vi "Host.vi"() -> ()   [LabVIEW 2019]
uses:
  <vilib>/Analysis/7linalg.llb/Eigenvalue and Vectors Output Option.ctl
  <vilib>/Analysis/baseanly.llb/Matrix Type of Inverse Matrix.ctl
  <vilib>/Analysis/7linalg.llb/Real Generalized Eigenvalues and Vectors.vi
  <vilib>/Analysis/7linalg.llb/Real Cholesky Factorization.vi
  <vilib>/Analysis/baseanly.llb/Full Cholesky Factorization.vi
  <vilib>/Analysis/baseanly.llb/Full Real Matrix Cholesky Factorization.vi
  <vilib>/FPGAPlugInAG/PXIe-7915/niLvFpga_Open_PXIe-7915.vi
  <vilib>/rvi/interface/common/dynamic/niFpgaDynamicAddResources.vi
  <vilib>/Analysis/baseanly.llb/Real Inverse Matrix.vi
  <vilib>/Analysis/Matrix/Numeric/Multiply/Multiply - RM,RM.vi
  <vilib>/Analysis/7linalg.llb/Real Eigenvalues and Vectors.vi
  <vilib>/Analysis/Matrix/Numeric/Add/Add - RM,RM.vi
  <vilib>/Utility/error.llb/Error Cluster From Error Code.vi
  <vilib>/rvi/errors/niLvFpgaAdjustHostInterfaceError.vi
  <vilib>/FPGAPlugInAG/Dynamic/niLvFpga_Run_Dynamic.vi
  <vilib>/FPGAPlugInAG/Dynamic/niLvFpga_Close_Dynamic.vi
  <vilib>/rvi/interface/nirviOpenFPGA/nirviOpenFPGA.xnode
  FPGA Bitfiles/choleskyfpgav1_FPGATarget_Target_xjOD3-+swO0.lvbitx
  Target.vi
  <vilib>/rvi/interface/nirviMethod/nirviMethod.xnode
  <vilib>/rvi/interface/nirviReadWriteControl/nirviReadWriteControl.xnode
  <vilib>/rvi/interface/nirviCloseFPGA/nirviCloseFPGA.xnode
  <vilib>/Analysis/NI_AALPro.lvlib
  <vilib>/Analysis/NI_AALBase.lvlib
  <vilib>/Analysis/Matrix/NI_Matrix.lvlib
  <vilib>/rvi/errors/niLvFpgaMergeErrorWithErrorCode.vi
  <vilib>/FPGAPlugInAG/Dynamic/niLvFpga_ReadFifo_Dynamic.vi
  <vilib>/FPGAPlugInAG/Dynamic/niLvFpga_WriteFifo_Dynamic.vi
  NiFpgaLv.dll
  <vilib>/rvi/interface/Simulation/niFpgaSimulationCallBeginRW.vi
panel:
  out "T5":u32
  out "T4":u32
  out "T3":u32
  out "T2":u32
  out "T1":u32
  out "Frequencies":dbl[](array[numeric])
  out "Eigenvalues":cdb[][](array[numeric]) format="%#_4g"
  out "Run Time (ms)":u32 format="%_6f"
  out "Elements Remaining 2":u32
  out "Elements Remaining":u32
  out "K input":dbl[][](array[numeric])
  in  "Method":i32(listbox)
  out "M input":dbl[][](array[numeric])
  # "Takes 56 ms to solve without timed loop"
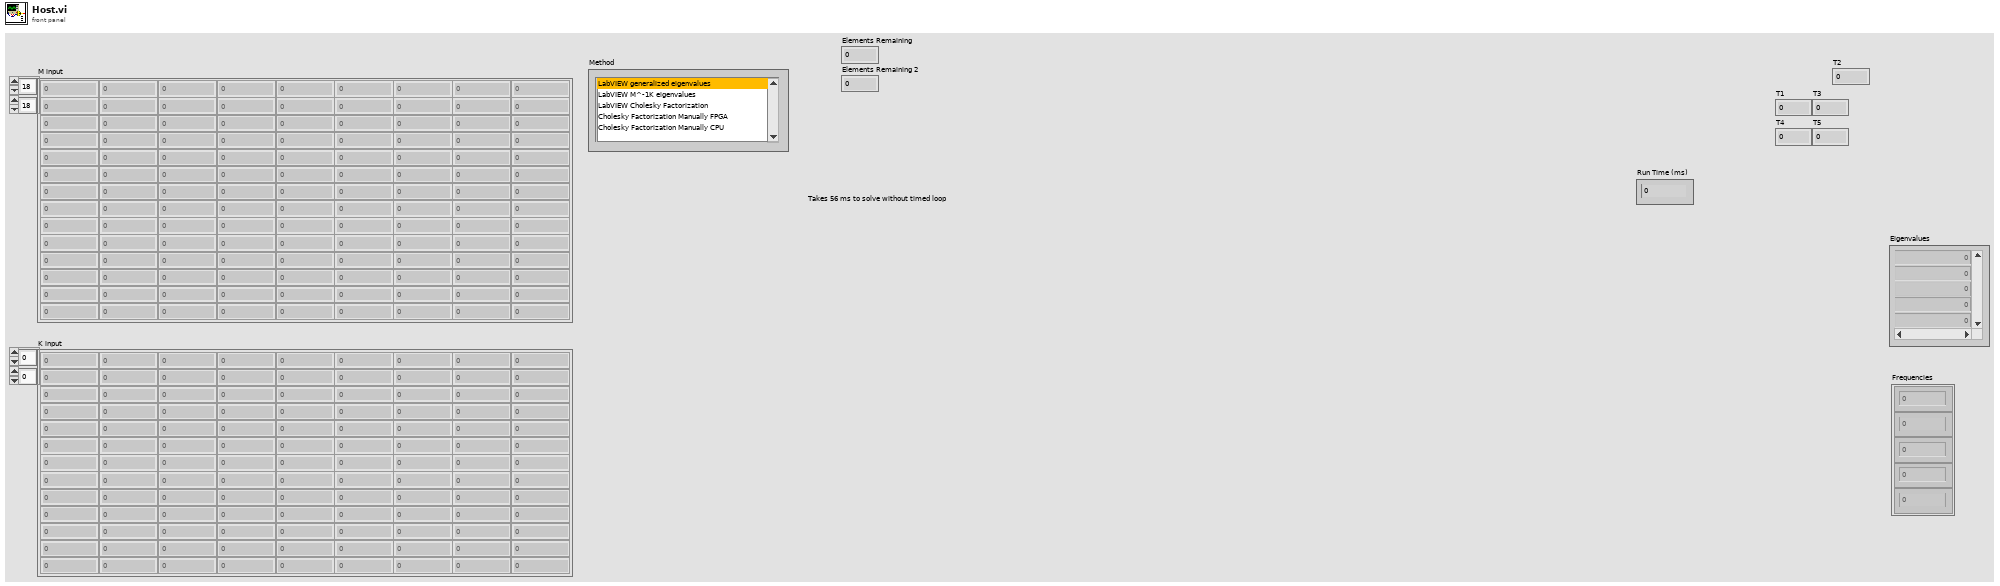
[diagram p1: front panel]
types:
  T1 = typedef "NI_AALBase.lvlib/Matrix Type of Inverse Matrix.ctl" = enum32{"General", "Positive Definite", "Lower Triangular", "Upper Triangular"}
  T2 = typedef "NI_AALPro.lvlib/Eigenvalue and Vectors Output Option.ctl" = i32
  T3 = typedef "NI_Matrix.lvlib/RealMatrix.ctl" = dbl[][]
  T4 = typedef "NI_Matrix.lvlib/ComplexMatrix.ctl" = cdb[][]
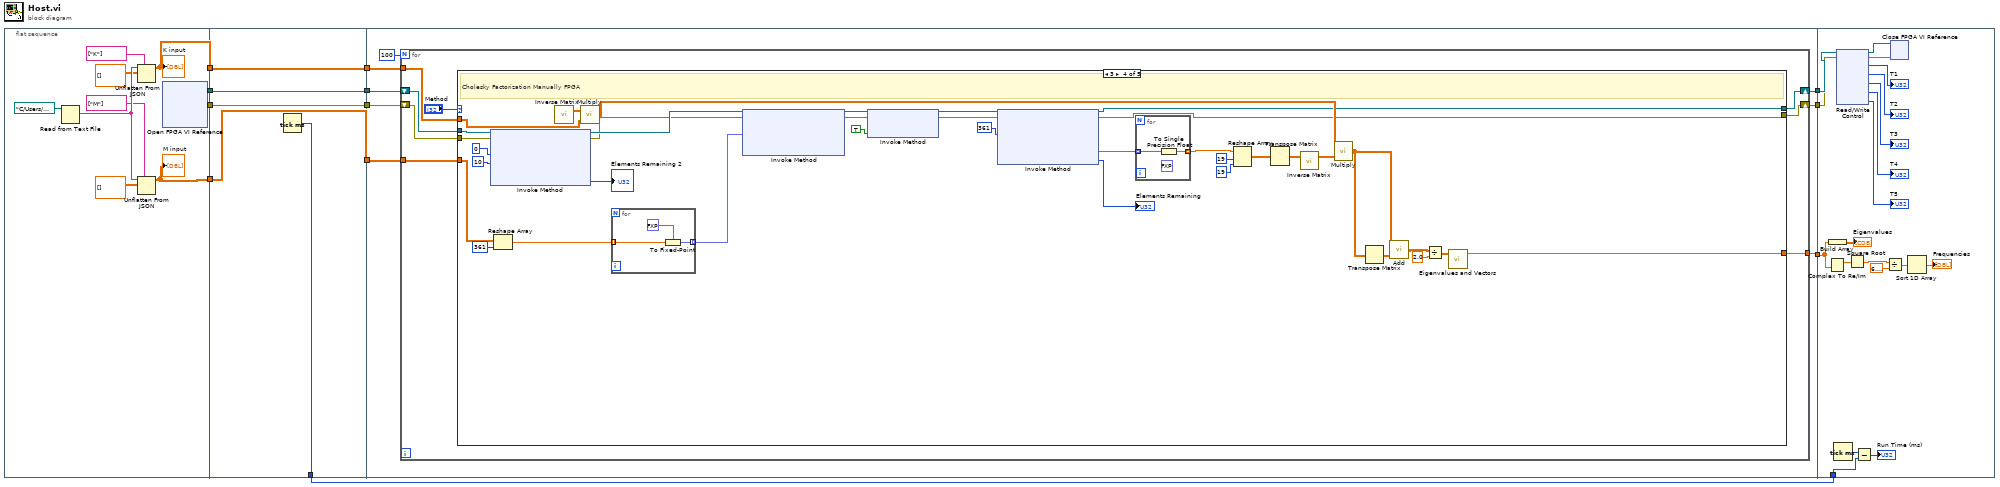
[diagram p0: block diagram]
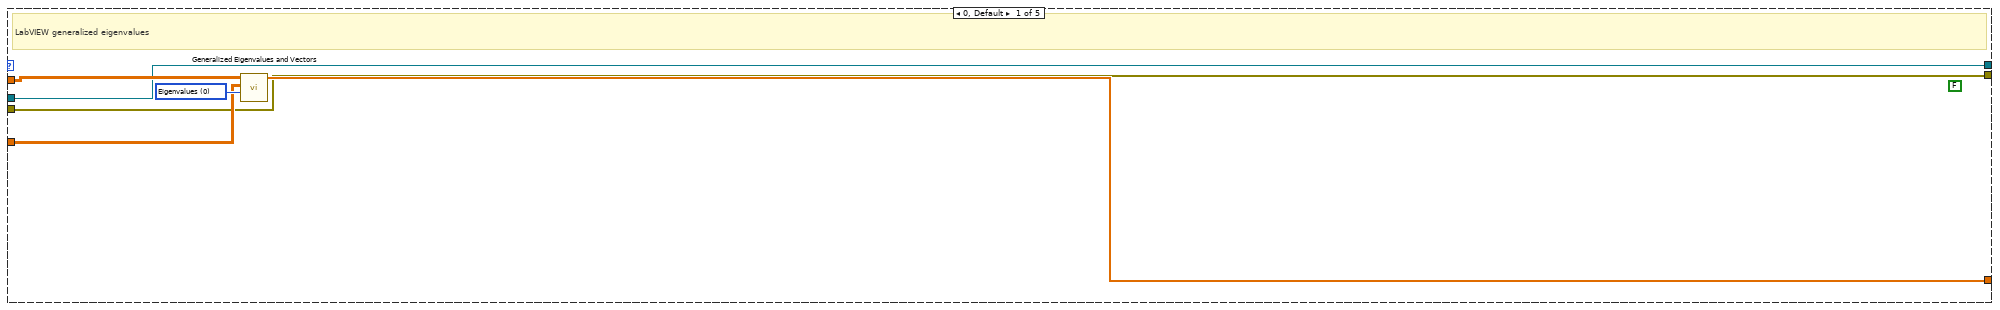
[diagram p2: hidden frame]
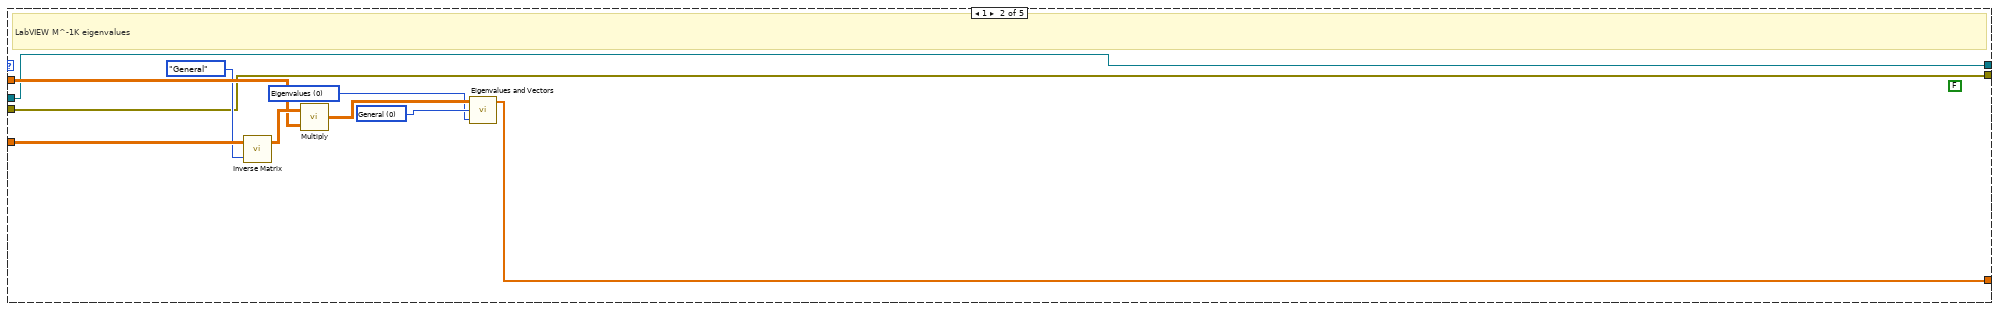
[diagram p3: hidden frame]
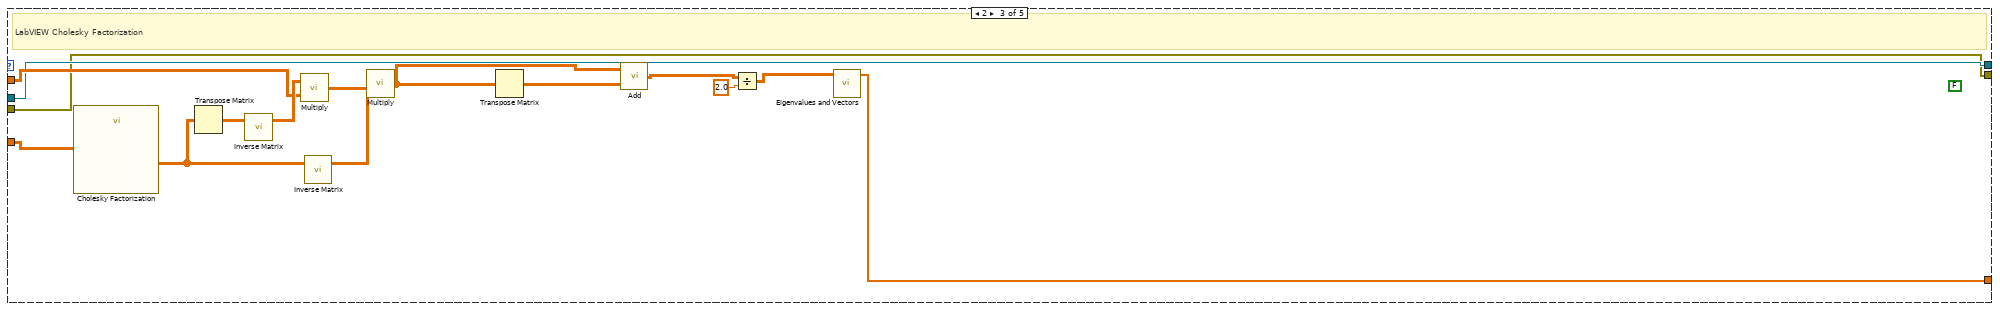
[diagram p4: hidden frame]
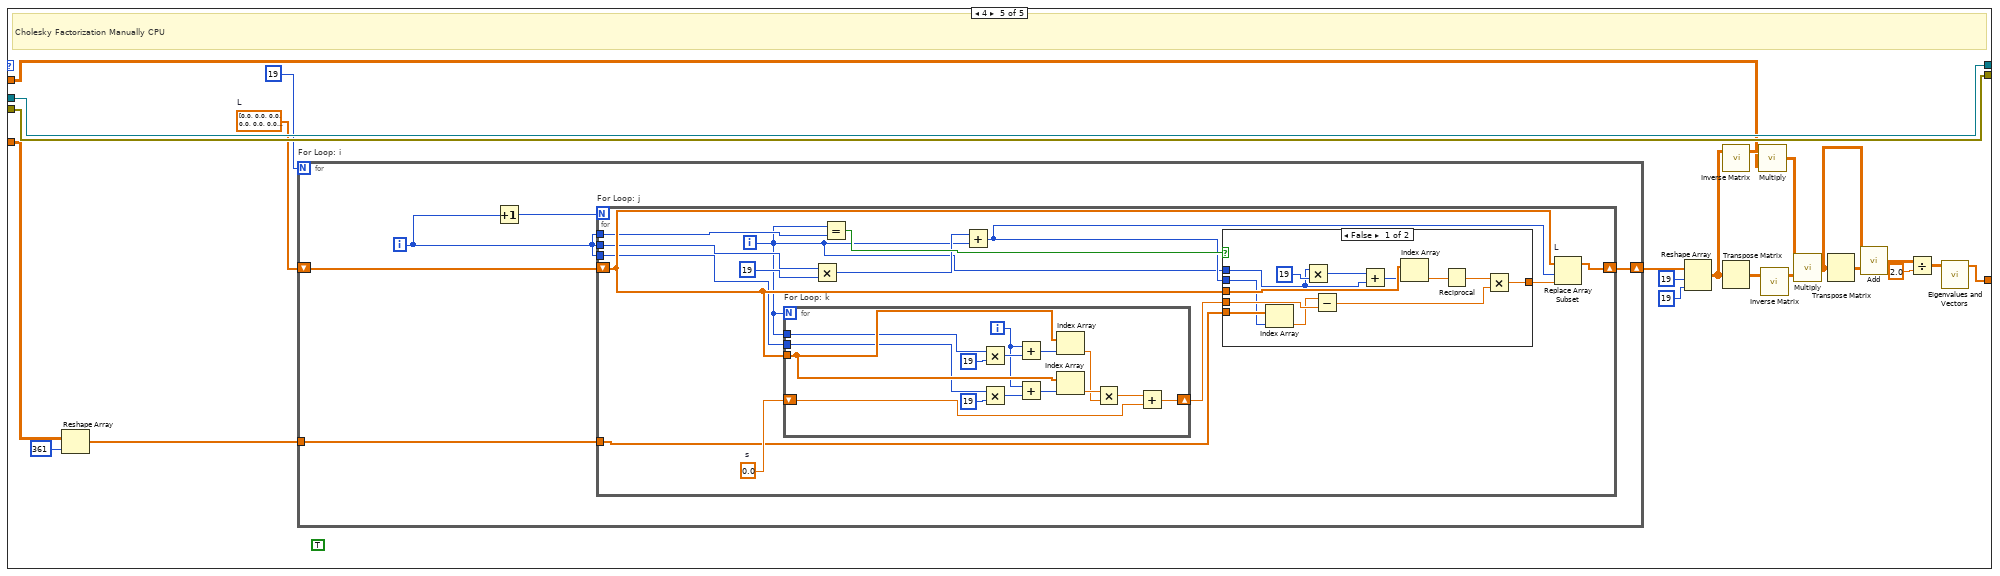
[diagram p5: hidden frame]
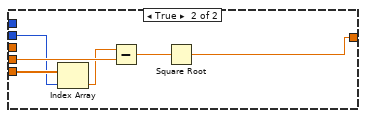
[diagram p6: hidden frame]
diagram:
  n1 = flat-sequence {
    tunnel: [w16] -> w10
    tunnel: [w15] -> w9
    tunnel: [w14] -> w7
    tunnel: [w13] -> w5
    tunnel: [w27] -> w12
    tunnel: [w26] -> w11
    tunnel: [w25] -> w1
    tunnel: w10 -> [w27]
    tunnel: w9 -> [w26]
    tunnel: [w24] -> w8
    tunnel: w7 -> [w24]
    tunnel: [w23] -> w6
    tunnel: w5 -> [w23]
    tunnel: w12 -> [w35]
    tunnel: w11 -> [w34]
    tunnel: w8 -> [w29]
    tunnel: w6 -> [w28]
    tunnel: [w33] -> w4
    tunnel: [w31] -> w3
    tunnel: [w30] -> w2
    tunnel: w4 -> [w196]
    tunnel: w3 -> [w195]
    tunnel: w2 -> [w194]
    tunnel: w1 -> [w193]
    frame #0 {
      n2 = Read from Text File(file (use dialog)=path "C:/Users/PXIe-8880/Documents/AFRL_summer_2019/Cholesky_FPGA/Cholesky_FPGA_V1/data/data.txt") -> (text=w22:string)  [unwired: 3 in, 3 out]
      n3 = Unflatten From JSON(path=string[] ["K"], JSON string=w22, type and defaults=dbl[][] []) -> (value=w15:dbl[][])  [unwired: 4 in, 1 out]
      "K input" <- w15
      n4 = Unflatten From JSON(path=string[] ["M"], JSON string=w22, type and defaults=dbl[][] []) -> (value=w16:dbl[][])  [unwired: 4 in, 1 out]
      "M input" <- w16
      n5 = xnode "Open FPGA VI Reference"() -> ("FPGA VI Reference Out"=w14:refnum<k20>, "error out"=w13:errorcluster)  [unwired: 2 in]
    }
    frame #1 {
      n6 = Tick Count (ms)() -> (millisecond timer value=w25:u32)
    }
    frame #2 {
      n7 = for {
        N: 100 -> [_]
        tunnel: w35 -> [w43]
        tunnel: w34 -> [w42]
        tunnel: [w39] -> w33
        shift-right: [w41] -> w31
        shift-left: w29 -> [w37]
        shift-right: [w40] -> w30
        shift-left: w28 -> [w36]
        n8 = case shown="3" "Method" {
          tunnel: [w48 w55 w68 w95 w116] -> w39
          tunnel: w43 -> [w47 w54 w74 w110 w117]
          tunnel: w42 -> [w46 w53 w70 w96 w118]
          tunnel: w37 -> [w45 w51 w61 w85 w137]
          tunnel: [w45 w51 w61 w89 w137] -> w41
          tunnel: w36 -> [w44 w50 w60 w84 w136]
          tunnel: [w44 w50 w60 w90 w136] -> w40
          frame 0, Default {
            (unwired) FALSE
            w49 = T2 0 items=["Eigenvalues", "Eigenvalues & Vectors"] ("output option")
            # "LabVIEW generalized eigenvalues"
            n9 = call-poly <vilib>:"Generalized Eigenvalues and Vectors.vi"("output option"=w49, "B"=w47, "A"=w46) -> ("Eigenvalues"=w48:cdb[])  [unwired: 3 in, 2 out]
          }
          frame 1 {
            (unwired) FALSE
            w56 = T2 0 items=["Eigenvalues", "Eigenvalues & Vectors"] ("output option")
            w57 = 0 items=["General", "Symmetric"] ("matrix type")
            # "LabVIEW M^-1K eigenvalues"
            n10 = call-poly <vilib>:"Inverse Matrix.vi"("matrix type"=Matrix_Type_of_Inverse_Matrix."General", "Input Matrix"=w54) -> ("Inverse Matrix"=w58:T3)  [unwired: 1 out]
            n11 = call-poly <vilib>:"Multiply.vi"("Real Matrix B"=w53, "Real Matrix A"=w58) -> ("A * B"=w59:T3)
            n12 = call-poly <vilib>:"Eigenvalues and Vectors.vi"("output option"=w56, "matrix type"=w57, "Input Matrix"=w59) -> ("Eigenvalues"=w55:cdb[])  [unwired: 2 out]
          }
          frame 2 {
            (unwired) FALSE
            # "LabVIEW Cholesky Factorization"
            n13 = call-poly <vilib>:"Cholesky Factorization.vi"("A"=w74) -> ("Cholesky"=w72:T3)  [unwired: 1 out]
            n14 = Transpose Matrix(1:w72) -> (0:w73:T3)
            n15 = call-poly <vilib>:"Inverse Matrix.vi"("Input Matrix"=w73) -> ("Inverse Matrix"=w71:T3)  [unwired: 1 in, 1 out]
            n16 = call-poly <vilib>:"Multiply.vi"("Real Matrix B"=w70, "Real Matrix A"=w71) -> ("A * B"=w67:T3)
            n17 = call-poly <vilib>:"Inverse Matrix.vi"("Input Matrix"=w72) -> ("Inverse Matrix"=w69:T3)  [unwired: 1 in, 1 out]
            n18 = call-poly <vilib>:"Multiply.vi"("Real Matrix B"=w69, "Real Matrix A"=w67) -> ("A * B"=w66:T3)
            n19 = Transpose Matrix(1:w66) -> (0:w65:T3)
            n20 = call-poly <vilib>:"Add.vi"("Real Matrix B"=w65, "Real Matrix A"=w66) -> ("A + B"=w63:T3)
            n21 = Divide(x=w63, y=2.0) -> (x/y=w62:T3)
            n22 = call-poly <vilib>:"Eigenvalues and Vectors.vi"("Input Matrix"=w62) -> ("Eigenvalues"=w68:cdb[])  [unwired: 2 in, 2 out]
          }
          frame 3 {
            # "Cholesky Factorization Manually FPGA"
            n23 = xnode "Invoke Method"("FPGA VI Reference In"=w85, "error in"=w84, "Number of Elements"=u32 0, "Timeout (ms)"=10) -> ("FPGA VI Reference Out"=w83:refnum<k20>, "error out"=w82:errorcluster, "Elements Remaining"=→"Elements Remaining 2":u32)  [unwired: 1 out]
            n24 = Reshape Array(w110, 361 ("dimension size")) -> (w79:dbl[])
            n25 = call-poly <vilib>:"Inverse Matrix.vi"() -> ("Inverse Matrix"=w105:T3)  [unwired: 2 in, 1 out]
            n26 = call-poly <vilib>:"Multiply.vi"("Real Matrix B"=w96, "Real Matrix A"=w105) -> ("A * B"=w103:T3)
            n27 = for {
              tunnel: w79 -> [w115] mode=indexing
              tunnel: [w114] -> w75 mode=indexing
              n28 = To Fixed-Point(fixed-point type=fxp<+/-,32,16> 0.0, number=w115) -> (fixed-point=w114:fxp<+/-,32,16>)
            }
            n29 = xnode "Invoke Method"("FPGA VI Reference In"=w83, "error in"=w82, "Data"=w75) -> ("FPGA VI Reference Out"=w94:refnum<k20>, "error out"=w93:errorcluster)  [unwired: 1 in, 1 out]
            n30 = xnode "Invoke Method"("FPGA VI Reference In"=w94, "error in"=w93, "Wait Until Done (F)"=TRUE) -> ("FPGA VI Reference Out"=w92:refnum<k20>, "error out"=w91:errorcluster)
            n31 = xnode "Invoke Method"("FPGA VI Reference In"=w92, "error in"=w91, "Number of Elements"=u32 361) -> ("FPGA VI Reference Out"=w89:refnum<k20>, "error out"=w90:errorcluster, "Data"=w78:fxp<+/-,32,0>[], "Elements Remaining"=→"Elements Remaining":u32)  [unwired: 1 in]
            n32 = for {
              tunnel: w78 -> [w112] mode=indexing
              tunnel: [w111] -> w77 mode=indexing
              (unwired) fxp<+/-,32,16> 0.0 ("fixed-point type")
              n33 = To Single Precision Float(number=w112) -> (single precision float=w111:sgl)
            }
            n34 = Reshape Array(w77, 19 ("dimension size"), 19 ("dimension size")) -> (w76:sgl[][])
            n35 = Transpose Matrix(1:w76) -> (0:w97:dbl[][])
            n36 = call-poly <vilib>:"Inverse Matrix.vi"("Input Matrix"=w97) -> ("Inverse Matrix"=w104:T3)  [unwired: 1 in, 1 out]
            n37 = call-poly <vilib>:"Multiply.vi"("Real Matrix B"=w104, "Real Matrix A"=w103) -> ("A * B"=w102:T3)
            n38 = Transpose Matrix(1:w102) -> (0:w101:T3)
            n39 = call-poly <vilib>:"Add.vi"("Real Matrix B"=w101, "Real Matrix A"=w102) -> ("A + B"=w99:T3)
            n40 = Divide(x=w99, y=2.0) -> (x/y=w98:T3)
            n41 = call-poly <vilib>:"Eigenvalues and Vectors.vi"("Input Matrix"=w98) -> ("Eigenvalues"=w95:cdb[])  [unwired: 2 in, 2 out]
          }
          frame 4 {
            w135 = sgl[] [0.0, 0.0, 0.0, 0.0, 0.0, 0.0, 0.0, 0.0, 0.0, 0.0, 0.0, 0.0, 0.0, 0.0, 0.0, 0.0, 0.0, 0.0, 0.0, 0.0, 0.0, 0.0, 0.0, 0.0, 0.0, 0.0, 0.0, 0.0, 0.0, 0.0, 0.0, 0.0, 0.0, 0.0, 0.0, 0.0, 0.0, 0.0, 0.0, 0.0, 0.0, 0.0, 0.0, 0.0, 0.0, 0.0, 0.0, 0.0, 0.0, 0.0, 0.0, 0.0, 0.0, 0.0, 0.0, 0.0, 0.0, 0.0, 0.0, 0.0, 0.0, 0.0, 0.0, 0.0, 0.0, 0.0, 0.0, 0.0, 0.0, 0.0, 0.0, 0.0, 0.0, 0.0, 0.0, 0.0, 0.0, 0.0, 0.0, 0.0, 0.0, 0.0, 0.0, 0.0, 0.0, 0.0, 0.0, 0.0, 0.0, 0.0, 0.0, 0.0, 0.0, 0.0, 0.0, 0.0, 0.0, 0.0, 0.0, 0.0, 0.0, 0.0, 0.0, 0.0, 0.0, 0.0, 0.0, 0.0, 0.0, 0.0, 0.0, 0.0, 0.0, 0.0, 0.0, 0.0, 0.0, 0.0, 0.0, 0.0, 0.0, 0.0, 0.0, 0.0, 0.0, 0.0, 0.0, 0.0, 0.0, 0.0, 0.0, 0.0, 0.0, 0.0, 0.0, 0.0, 0.0, 0.0, 0.0, 0.0, 0.0, 0.0, 0.0, 0.0, 0.0, 0.0, 0.0, 0.0, 0.0, 0.0, 0.0, 0.0, 0.0, 0.0, 0.0, 0.0, 0.0, 0.0, 0.0, 0.0, 0.0, 0.0, 0.0, 0.0, 0.0, 0.0, 0.0, 0.0, 0.0, 0.0, 0.0, 0.0, 0.0, 0.0, 0.0, 0.0, 0.0, 0.0, 0.0, 0.0, 0.0, 0.0, 0.0, 0.0, 0.0, 0.0, 0.0, 0.0, 0.0, 0.0, 0.0, 0.0, 0.0, 0.0, 0.0, 0.0, 0.0, 0.0, 0.0, 0.0, 0.0, 0.0, 0.0, 0.0, 0.0, 0.0, 0.0, 0.0, 0.0, 0.0, 0.0, 0.0, 0.0, 0.0, 0.0, 0.0, 0.0, 0.0, 0.0, 0.0, 0.0, 0.0, 0.0, 0.0, 0.0, 0.0, 0.0, 0.0, 0.0, 0.0, 0.0, 0.0, 0.0, 0.0, 0.0, 0.0, 0.0, 0.0, 0.0, 0.0, 0.0, 0.0, 0.0, 0.0, 0.0, 0.0, 0.0, 0.0, 0.0, 0.0, 0.0, 0.0, 0.0, 0.0, 0.0, 0.0, 0.0, 0.0, 0.0, 0.0, 0.0, 0.0, 0.0, 0.0, 0.0, 0.0, 0.0, 0.0, 0.0, 0.0, 0.0, 0.0, 0.0, 0.0, 0.0, 0.0, 0.0, 0.0, 0.0, 0.0, 0.0, 0.0, 0.0, 0.0, 0.0, 0.0, 0.0, 0.0, 0.0, 0.0, 0.0, 0.0, 0.0, 0.0, 0.0, 0.0, 0.0, 0.0, 0.0, 0.0, 0.0, 0.0, 0.0, 0.0, 0.0, 0.0, 0.0, 0.0, 0.0, 0.0, 0.0, 0.0, 0.0, 0.0, 0.0, 0.0, 0.0, 0.0, 0.0, 0.0, 0.0, 0.0, 0.0, 0.0, 0.0, 0.0, 0.0, 0.0, 0.0, 0.0, 0.0, 0.0, 0.0, 0.0, 0.0, 0.0, 0.0, 0.0, 0.0, 0.0, 0.0, 0.0, 0.0, 0.0, 0.0, 0.0, 0.0, 0.0, 0.0, 0.0, 0.0, 0.0, 0.0, 0.0, 0.0, 0.0, 0.0, 0.0, 0.0, 0.0, 0.0]  # L
            (unwired) TRUE
            # "Cholesky Factorization Manually CPU"
            n42 = Reshape Array(w117, 361 ("dimension size")) -> (w132:dbl[])
            n43 = for "For Loop: i" {
              N: 19 -> [_]
              shift-right: [w140] -> w120
              shift-left: w135 -> [w142]
              tunnel: w132 -> [w139]
              i -> [w138]
              n44 = Increment(x=w138) -> (x+1=w141:i32)
              n45 = for "For Loop: j" {
                N: w141 -> [_]
                tunnel: w138 -> [w150]
                shift-right: [w152] -> w140
                shift-left: w142 -> [w151]
                tunnel: w138 -> [w149]
                tunnel: w139 -> [w146]
                tunnel: w138 -> [w144]
                i -> [w143]
                w155 = sgl 0.0  # s
                n46 = for "For Loop: k" {
                  N: w143 -> [_]
                  tunnel: w151 -> [w189]
                  shift-right: [w185] -> w154
                  shift-left: w155 -> [w186]
                  tunnel: w144 -> [w184]
                  tunnel: w143 -> [w177]
                  i -> [w176]
                  n47 = Multiply(x=w177, y=19) -> (x*y=w179:i32)
                  n48 = Multiply(x=w184, y=19) -> (x*y=w182:i32)
                  n49 = Add(x=w176, y=w179) -> (x+y=w178:i32)
                  n50 = Add(x=w176, y=w182) -> (x+y=w181:i32)
                  n51 = Index Array(array=w189, index=w178) -> (element=w188:sgl)
                  n52 = Index Array(array=w189, index=w181) -> (element=w190:sgl)
                  n53 = Multiply(x=w190, y=w188) -> (x*y=w187:sgl)
                  n54 = Add(x=w187, y=w186) -> (x+y=w185:sgl)
                }
                n55 = Multiply(x=w149, y=19) -> (x*y=w147:i32)
                n56 = Equal?(x=w143, y=w150) -> (x = y?=w156:bool)
                n57 = Add(x=w147, y=w143) -> (x+y=w145:i32)
                n58 = case shown="False" w156 {
                  tunnel: w154 -> [w167 w175]
                  tunnel: [w166 w173] -> w153
                  tunnel: w151 -> [w169 _]
                  tunnel: w146 -> [w163 w172]
                  tunnel: w145 -> [w162 w171]
                  tunnel: w143 -> [w158 _]
                  frame False {
                    n59 = Index Array(array=w163, index=w162) -> (element=w161:dbl)
                    n60 = Multiply(x=w158, y=19) -> (x*y=w159:i32)
                    n61 = Subtract(x=w161, y=w167) -> (x-y=w164:dbl)
                    n62 = Add(x=w159, y=w158) -> (x+y=w157:i32)
                    n63 = Index Array(array=w169, index=w157) -> (element=w168:sgl)
                    n64 = Reciprocal(x=w168) -> (1/x=w165:sgl)
                    n65 = Multiply(x=w165, y=w164) -> (x*y=w166:dbl)
                  }
                  frame True {
                    n66 = Index Array(array=w172, index=w171) -> (element=w170:dbl)
                    n67 = Subtract(x=w170, y=w175) -> (x-y=w174:dbl)
                    n68 = Square Root(x=w174) -> (sqrt(x)=w173:dbl)
                  }
                }
                n69 = Replace Array Subset "L"(array=w151, new element=w153, index=w145) -> (w152:sgl[])
              }
            }
            n70 = Reshape Array(w120, 19 ("dimension size"), 19 ("dimension size")) -> (w119:sgl[][])
            n71 = call-poly <vilib>:"Inverse Matrix.vi"("Input Matrix"=w119) -> ("Inverse Matrix"=w129:T3)  [unwired: 1 in, 1 out]
            n72 = Transpose Matrix(1:w119) -> (0:w121:dbl[][])
            n73 = call-poly <vilib>:"Multiply.vi"("Real Matrix B"=w118, "Real Matrix A"=w129) -> ("A * B"=w127:T3)
            n74 = call-poly <vilib>:"Inverse Matrix.vi"("Input Matrix"=w121) -> ("Inverse Matrix"=w128:T3)  [unwired: 1 in, 1 out]
            n75 = call-poly <vilib>:"Multiply.vi"("Real Matrix B"=w128, "Real Matrix A"=w127) -> ("A * B"=w126:T3)
            n76 = Transpose Matrix(1:w126) -> (0:w125:T3)
            n77 = call-poly <vilib>:"Add.vi"("Real Matrix B"=w125, "Real Matrix A"=w126) -> ("A + B"=w123:T3)
            n78 = Divide(x=w123, y=2.0) -> (x/y=w122:T3)
            n79 = call-poly <vilib>:"Eigenvalues and Vectors.vi"("Input Matrix"=w122) -> ("Eigenvalues"=w116:cdb[])  [unwired: 2 in, 2 out]
          }
        }
      }
    }
    frame #3 {
      n80 = Build Array(w196) -> (→"Eigenvalues":T4)
      n81 = Complex To Re/Im ("Complex To Cartesian.vi")(x + iy=w196) -> (x=w207:dbl[])  [unwired: 1 out]
      n82 = Tick Count (ms)() -> (millisecond timer value=w192:u32)
      n83 = xnode "Read/Write Control"("FPGA VI Reference In"=w195, "error in"=w194) -> ("FPGA VI Reference Out"=w203:refnum<k20>, "error out"=w202:errorcluster, "T1"=→"T1":u32, "T2"=→"T2":u32, "T3"=→"T3":u32, "T4"=→"T4":u32, "T5"=→"T5":u32)
      n84 = Square Root ("Square Root.vi")(x=w207) -> (sqrt(x)=w208:dbl[])
      n85 = Subtract(x=w192, y=w193) -> (x-y=→"Run Time (ms)":u32)
      n86 = Divide(x=w208, y=6.283185307179586) -> (x/y=w209:dbl[])
      n87 = xnode "Close FPGA VI Reference"("FPGA VI Reference In"=w203, "error in"=w202) -> ()  [unwired: 1 out]
      n88 = Sort 1D Array(array=w209) -> (sorted array=→"Frequencies":dbl[])
    }
  }
